vi "BLE_StartWatcher.vi"(0 ".NET Refnum in":refnum<k24>, 11 "error in (no error)":errorcluster) -> (4 ".NET Refnum out":refnum<k24>, 6 "StartDeviceWatcher":string, 15 "error out":errorcluster)   [LabVIEW 2020]
uses:
  C:/Users/bharathi.t/Downloads/Bluetooth - Copy/Bluetooth/BLE/BLELib.dll
  BLELib.dll
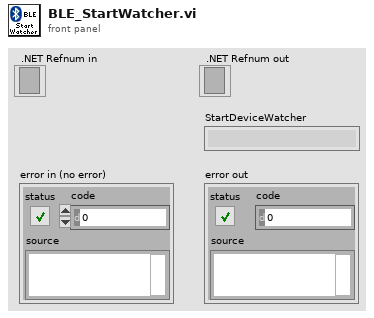
[diagram p1: front panel]
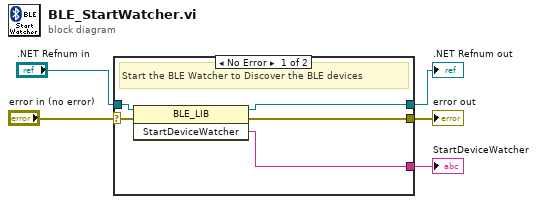
[diagram p0: block diagram]
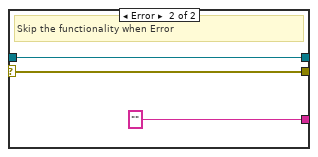
[diagram p2: hidden frame]
diagram:
  n1 = case shown="No Error" "error in (no error)" {
    selector: "error in (no error)" -> [w7 w12]
    tunnel: [w10 w12] -> w5
    tunnel: [w9 w13] -> w4
    tunnel: [w8 "" ("StartDeviceWatcher")] -> w3
    tunnel: ".NET Refnum in" -> [w6 w13]
    frame No Error {
      # "Start the BLE Watcher to Discover the BLE devices"
      n2 = invoke class="BLE_LIB" method="StartDeviceWatcher"(reference=w6, error in=w7) -> (reference out=w9:refnum<k24>, error out=w10:errorcluster, "StartDeviceWatcher"=w8:string)  [unwired: 1 in]
    }
    frame Error {
      # "Skip the functionality when Error"
    }
  }
  "StartDeviceWatcher" <- w3
  "error out" <- w5
  ".NET Refnum out" <- w4
